vi "TODO Variant data to time series JSON data.vi"(8 "error in (no error)":errorcluster, 9 "Precision":T1=enum."Nanoseconds", 10 "Data":variant, 11 "Series name":string="testSeries") -> (0 "error out":errorcluster, 3 "JSON data":string="[{\"name\":\"testSeries\",\"columns\":[[\"time\",\"host\",\"value\"]],\"points\":[[[1430144955,\"serverA\",\" 23.299999\"],[1429280957,\"serverB\",\" 24.5\"]]]}]")   [LabVIEW 2018, in "InfluxDB Client.lvlib" / "Client.lvclass"]
doc: "Convert variant data (cluster with one ore more controls) to time series JSON data."
uses:
  Client.lvclass
  Controls/Precision.ctl
  <vilib>/Utility/VariantDataType/VariantType.lvlib
  InfluxDB Client.lvlib
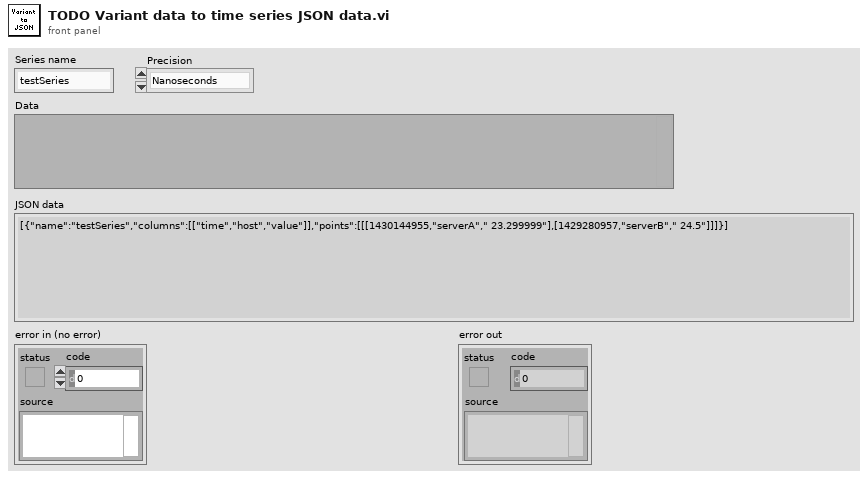
[diagram p1: front panel]
types:
  T1 = typedef "InfluxDB Client.lvlib/Precision.ctl" = enum16{"Seconds", "Milliseconds", "Nanoseconds"}
  T2 = typedef "VariantType.lvlib/Type.ctl" = enum8{"Invalid Type", "Void", "I8", "I16", "I32", "I64", "U8", "U16", "U32", "U64", "Single Float", "Double Float", "Extended Float", "Single Complex", "Double Complex", "Extended Complex", "Enum U8", "Enum U16", "Enum U32", "Enum U64", "Single Float With Unit", "Double Float With Unit", "Extended Float With Unit", "Single Complex with Unit", "Double Complex with Unit", "Extended Complex with Unit", "Boolean", "String", "Path", "Picture", "Tag", "Array", "Cluster", "Variant", "LV Variant", "Waveform", "Timestamp", "Digital Waveform", "Digital Data", "ExpressData", "Refnum", "External Data", "VI", "Poly VI", "LabVIEW Class Instance", "Fixed Point"}
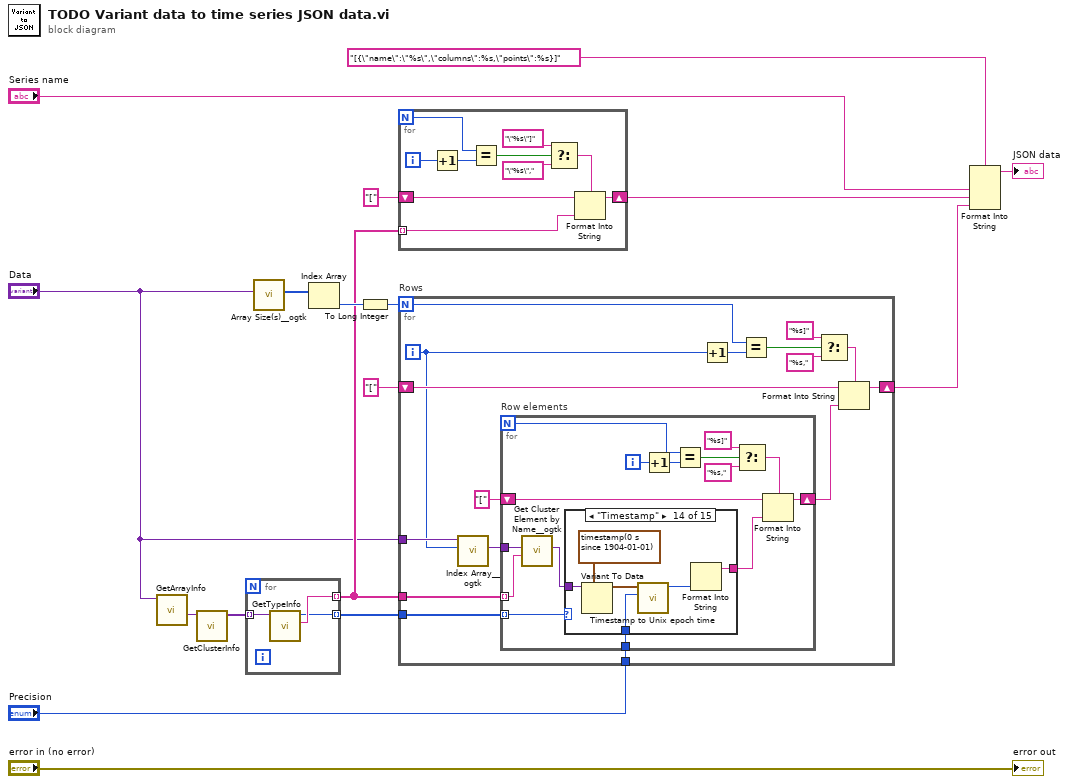
[diagram p0: block diagram]
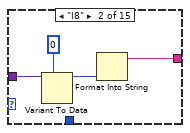
[diagram p3: hidden frame]
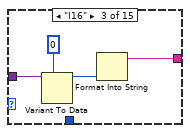
[diagram p4: hidden frame]
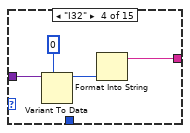
[diagram p5: hidden frame]
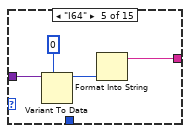
[diagram p6: hidden frame]
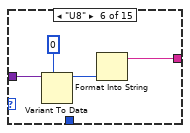
[diagram p7: hidden frame]
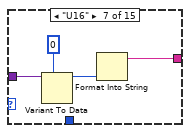
[diagram p8: hidden frame]
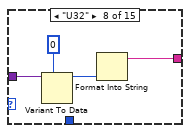
[diagram p9: hidden frame]
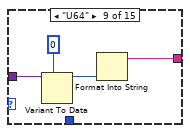
[diagram p10: hidden frame]
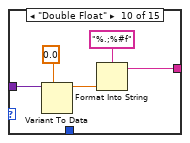
[diagram p11: hidden frame]
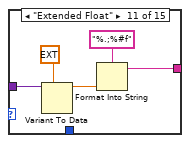
[diagram p12: hidden frame]
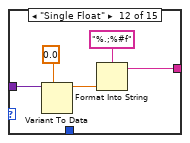
[diagram p13: hidden frame]
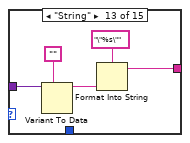
[diagram p14: hidden frame]
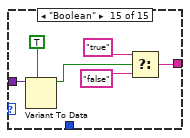
[diagram p15: hidden frame]
diagram:
  n1 = call <vilib>:"GetArrayInfo.vi"("Variant"="Data") -> ("ArrayElement"=w12:variant)  [unwired: 7 in, 3 out]
  n2 = call <vilib>:"GetClusterInfo.vi"("Variant"=w12) -> ("Cluster Elements"=w11:variant[])  [unwired: 9 in, 1 out]
  n3 = for {
    tunnel: [w19] -> w6 mode=indexing
    tunnel: [w20] -> w4 mode=indexing
    tunnel: w11 -> [w18] mode=indexing
    n4 = call <vilib>:"GetTypeInfo.vi"("Variant"=w18) -> ("Name"=w20:string, "Type Enum"=w19:T2)  [unwired: 6 in, 3 out]
  }
  n5 = call <userlib>:"Array Size(s)__ogtk.vi"("Array"="Data") -> ("Size(s)"=w10:u32[])  [unwired: 8 in, 2 out]
  n6 = Index Array(array=w10) -> (element=w9:u32)  [unwired: 1 in]
  n7 = To Long Integer(number=w9) -> (32bit integer=w7:i32)
  n8 = for {
    N -> [w22]
    tunnel: w4 -> [w29] mode=indexing
    shift-right: [w30] -> w16
    shift-left: "[" -> [w28]
    i -> [w24]
    n9 = Increment(x=w24) -> (x+1=w23:i32)
    n10 = Equal?(x=w22, y=w23) -> (x = y?=w21:bool)
    n11 = Select(t="\"%s\"]" ("format string"), s=w21, f="\"%s\"," ("format string")) -> (s? t:f=w25:string)
    n12 = Format Into String(format string=w25, initial string=w28, w29) -> (resulting string=w30:string)  [unwired: 1 in, 1 out]
  }
  n13 = for "Rows" {
    N: w7 -> [w39]
    tunnel: w4 -> [w46]
    tunnel: w6 -> [w45]
    shift-right: [w37] -> w5
    shift-left: "[" -> [w38]
    tunnel: "Data" -> [w34]
    tunnel: "Precision" -> [w31]
    i -> [w33]
    n14 = call <userlib>:"Index Array__ogtk.vi"("Index (1D)"=w33, "MultiD Array"=w34) -> ("Array Element"=w32:variant)  [unwired: 8 in, 1 out]
    n15 = for "Row elements" {
      N -> [w53]
      tunnel: w32 -> [w61]
      tunnel: w46 -> [w60] mode=indexing
      tunnel: w45 -> [w58] mode=indexing
      shift-right: [w50] -> w35
      shift-left: "[" -> [w48]
      tunnel: w31 -> [w47]
      i -> [w52]
      n16 = call <userlib>:"Get Cluster Element by Name__ogtk.vi"("Element Name"=w60, "Cluster"=w61) -> ("VElement"=w59:variant)  [unwired: 7 in, 2 out]
      n17 = case shown="\"Timestamp\"" w58 {
        tunnel: w59 -> [_ w64 w68 w72 w76 w80 w84 w88 w92 w97 w102 w107 w112 w119 w125]
        tunnel: [_ w62 w66 w70 w74 w78 w82 w86 w90 w95 w100 w105 w110 w115 w123] -> w49
        tunnel: w47 -> [_ _ _ _ _ _ _ _ _ _ _ _ _ w114 _]
        frame Default {
          # "todo assert"
        }
        frame "I8" {
          n18 = Variant To Data(type=i8 0, Variant=w64) -> (data=w63:i8)  [unwired: 1 in, 1 out]
          n19 = Format Into String(w63) -> (resulting string=w62:string)  [unwired: 3 in, 1 out]
        }
        frame "I16" {
          n20 = Variant To Data(type=i16 0, Variant=w68) -> (data=w67:i16)  [unwired: 1 in, 1 out]
          n21 = Format Into String(w67) -> (resulting string=w66:string)  [unwired: 3 in, 1 out]
        }
        frame "I32" {
          n22 = Variant To Data(type=0, Variant=w72) -> (data=w71:i32)  [unwired: 1 in, 1 out]
          n23 = Format Into String(w71) -> (resulting string=w70:string)  [unwired: 3 in, 1 out]
        }
        frame "I64" {
          n24 = Variant To Data(type=i64 0, Variant=w76) -> (data=w75:i64)  [unwired: 1 in, 1 out]
          n25 = Format Into String(w75) -> (resulting string=w74:string)  [unwired: 3 in, 1 out]
        }
        frame "U8" {
          n26 = Variant To Data(type=u8 0, Variant=w80) -> (data=w79:u8)  [unwired: 1 in, 1 out]
          n27 = Format Into String(w79) -> (resulting string=w78:string)  [unwired: 3 in, 1 out]
        }
        frame "U16" {
          n28 = Variant To Data(type=u16 0, Variant=w84) -> (data=w83:u16)  [unwired: 1 in, 1 out]
          n29 = Format Into String(w83) -> (resulting string=w82:string)  [unwired: 3 in, 1 out]
        }
        frame "U32" {
          n30 = Variant To Data(type=u32 0, Variant=w88) -> (data=w87:u32)  [unwired: 1 in, 1 out]
          n31 = Format Into String(w87) -> (resulting string=w86:string)  [unwired: 3 in, 1 out]
        }
        frame "U64" {
          n32 = Variant To Data(type=u64 0, Variant=w92) -> (data=w91:u64)  [unwired: 1 in, 1 out]
          n33 = Format Into String(w91) -> (resulting string=w90:string)  [unwired: 3 in, 1 out]
        }
        frame "Double Float" {
          n34 = Variant To Data(type=0.0, Variant=w97) -> (data=w96:dbl)  [unwired: 1 in, 1 out]
          n35 = Format Into String(format string="%.;%#f", w96) -> (resulting string=w95:string)  [unwired: 2 in, 1 out]
        }
        frame "Extended Float" {
          n36 = Variant To Data(type=ext 0.0, Variant=w102) -> (data=w101:ext)  [unwired: 1 in, 1 out]
          n37 = Format Into String(format string="%.;%#f", w101) -> (resulting string=w100:string)  [unwired: 2 in, 1 out]
        }
        frame "Single Float" {
          n38 = Variant To Data(type=sgl 0.0, Variant=w107) -> (data=w106:sgl)  [unwired: 1 in, 1 out]
          n39 = Format Into String(format string="%.;%#f", w106) -> (resulting string=w105:string)  [unwired: 2 in, 1 out]
        }
        frame "String" {
          n40 = Variant To Data(type="", Variant=w112) -> (data=w111:string)  [unwired: 1 in, 1 out]
          n41 = Format Into String(format string="\"%s\"", w111) -> (resulting string=w110:string)  [unwired: 2 in, 1 out]
        }
        frame "Timestamp" {
          n42 = Variant To Data(type=timestamp(0 s since 1904-01-01), Variant=w119) -> (data=w118:timestamp)  [unwired: 1 in, 1 out]
          n43 = call "Timestamp to Unix epoch time.vi"("Precision (ns)"=w114, "Timestamp"=w118) -> ("Unix epoch time"=w116:u64)  [unwired: 9 in]
          n44 = Format Into String(w116) -> (resulting string=w115:string)  [unwired: 3 in, 1 out]
        }
        frame "Boolean" {
          n45 = Variant To Data(type=TRUE, Variant=w125) -> (data=w120:bool)  [unwired: 1 in, 1 out]
          n46 = Select(t="true" ("format string"), s=w120, f="false" ("format string")) -> (s? t:f=w123:string)
        }
      }
      n47 = Increment(x=w52) -> (x+1=w56:i32)
      n48 = Equal?(x=w53, y=w56) -> (x = y?=w57:bool)
      n49 = Select(t="%s]" ("format string"), s=w57, f="%s," ("format string")) -> (s? t:f=w51:string)
      n50 = Format Into String(format string=w51, initial string=w48, w49) -> (resulting string=w50:string)  [unwired: 1 in, 1 out]
    }
    n51 = Increment(x=w33) -> (x+1=w41:i32)
    n52 = Equal?(x=w39, y=w41) -> (x = y?=w40:bool)
    n53 = Select(t="%s]" ("format string"), s=w40, f="%s," ("format string")) -> (s? t:f=w36:string)
    n54 = Format Into String(format string=w36, initial string=w38, w35) -> (resulting string=w37:string)  [unwired: 1 in, 1 out]
  }
  n55 = Format Into String(format string="[{\"name\":\"%s\",\"columns\":%s,\"points\":%s}]", "Series name", w16, w5) -> (resulting string=→"JSON data":string)  [unwired: 2 in, 1 out]
  "error out" <- "error in (no error)"
